vi "Teleop.vi"(10 "Match Info":T1={"Autonomous Elapsed Seconds"=0.0, "TeleOp Elapsed Seconds"=0.0, "Disabled Elapsed Seconds"=0.0, "Visited Autonomous"=FALSE, "Visited TeleOp"=FALSE, "Visited Disabled"=FALSE, "Autonomous Settings"={"Autonomous Style"=enum."Independent", "VI Refnum"=refnum}}, 11 "Call Context":T2) -> ()   [LabVIEW 2015]
doc: "This VI is called for each TeleOp packet received from the DS where the robot is not disabled. It is often used to read from the joysticks and update I/O or to update setpoints for timed control loops. It should complete and return within 20 milliseconds or it may miss DS packets."
uses:
  <vilib>/Rock Robotics/WPI/DriverStation/WPI_DriverStationDerivedRobotMode.ctl
  <vilib>/Rock Robotics/WPI/DriverStation/WPI_DriverStationMatch Info.ctl
  <vilib>/Rock Robotics/WPI/Utilities/WPI_GetSetVariantRefNum.vi
  <vilib>/Rock Robotics/Network Tables/NT Write Boolean Array.vi
  <vilib>/Rock Robotics/Network Tables/NT Write Numeric Array.vi
  <vilib>/Rock Robotics/Network Tables/NT Read Boolean.vi
  <vilib>/Rock Robotics/Network Tables/NT Read Number.vi
panel:
  out "Sample Slider 0":dbl(slide) scale=0.0..5.0
  out "Sample Boolean 1":bool
  out "Sample Boolean 0":bool
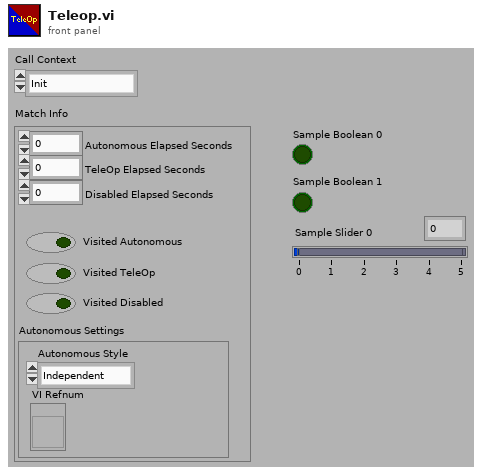
[diagram p1: front panel]
types:
  T1 = typedef "WPI_DriverStationMatch Info.ctl" = cluster{"Autonomous Elapsed Seconds":dbl, "TeleOp Elapsed Seconds":dbl, "Disabled Elapsed Seconds":dbl, "Visited Autonomous":bool, "Visited TeleOp":bool, "Visited Disabled":bool, "Autonomous Settings":cluster{"Autonomous Style":enum16{"Iterative", "Independent"}, "VI Refnum":refnum<vi>}}
  T2 = typedef "WPI_DriverStationDerivedRobotMode.ctl" = enum16{"Init", "Execute", "Stop"}
  T3 = typedef "WPI_JoystickDevRef.ctl" = cluster{"Device":T4}
  T4 = typedef "WPI_JoystickDeviceEnum.ctl" = enum16{"USB 0", "USB 1", "USB 2", "USB 3", "USB 4", "USB 5"}
  T5 = typedef "WPI_RobotDriveDevRef.ctl" = cluster{"DevStatus":errorcluster, "Motors[]":T6[], "Square Inputs":bool, "Max Output":dbl}
  T6 = typedef "WPI_MotorControlDeviceRef.ctl" = cluster{"DeviceStatus":errorcluster, "Type":T7, "PWM":cluster{"PWM Channel":T8, "DeadBand":T9}, "CAN":cluster{"Device Number":u8, "Control Mode":T10, "Semaphore":T11, "Max Vout":dbl, "TalonSRX Control Mode":T12}, "Invert":bool}
  T7 = typedef "WPI_MotorControlType.ctl" = enum16{"PWM", "CAN", "CANTalonSRX"}
  T8 = typedef "FPGA_DIOPWMChannel.ctl" = enum8{"PWM 0", "PWM 1", "PWM 2", "PWM 3", "PWM 4", "PWM 5", "PWM 6", "PWM 7", "PWM 8", "PWM 9", "PWM MXP 0", "PWM MXP 1", "PWM MXP 2", "PWM MXP 3", "PWM MXP 4", "PWM MXP 5", "PWM MXP 6", "PWM MXP 7", "PWM MXP 8", "PWM MXP 9", "Invalid"}
  T9 = typedef "WPI_PWMDeadband.ctl" = cluster{"Name":string, "maxPositivePwm":i32, "minPositivePwm":i32, "centerPwm":i32, "maxNegativePwm":i32, "minNegativePwm":i32, "angularRange":u16}
  T10 = typedef "WPI_CANJaguar_ControlMode.ctl" = enum8{"Percent VBus", "Current", "Speed", "Position", "Voltage"}
  T11 = typedef "Semaphore RefNum" = refnum<k1>
  T12 = typedef "WPI_CANTalonSRX_APIControlMode.ctl" = enum8{"Percent VBus", "Speed", "Position", "Slave", "Unchanged / Invalid", "Voltage Compensation", "Current", "Motion Profile"}
  T13 = typedef "WPI_SwitchDevRef.ctl" = cluster{"DevStatus":errorcluster, "DIO Channel":T14, "CntIndex":T15, "Normally Closed":bool}
  T14 = typedef "FPGA_DIOChannel.ctl" = enum8{"DIO 0", "DIO 1", "DIO 2", "DIO 3", "DIO 4", "DIO 5", "DIO 6", "DIO 7", "DIO 8", "DIO 9", "DIO MXP 0", "DIO MXP 1", "DIO MXP 2", "DIO MXP 3", "DIO MXP 4", "DIO MXP 5", "DIO MXP 6", "DIO MXP 7", "DIO MXP 8", "DIO MXP 9", "DIO MXP 10", "DIO MXP 11", "DIO MXP 12", "DIO MXP 13", "DIO MXP 14", "DIO MXP 15", "Invalid"}
  T15 = typedef "FPGA_CounterCtrSystemIndex.ctl" = enum8{"Ctr 0", "Ctr 1", "Ctr 2", "Ctr 3", "Ctr 4", "Ctr 5", "Ctr 6", "Ctr 7", "Invalid"}
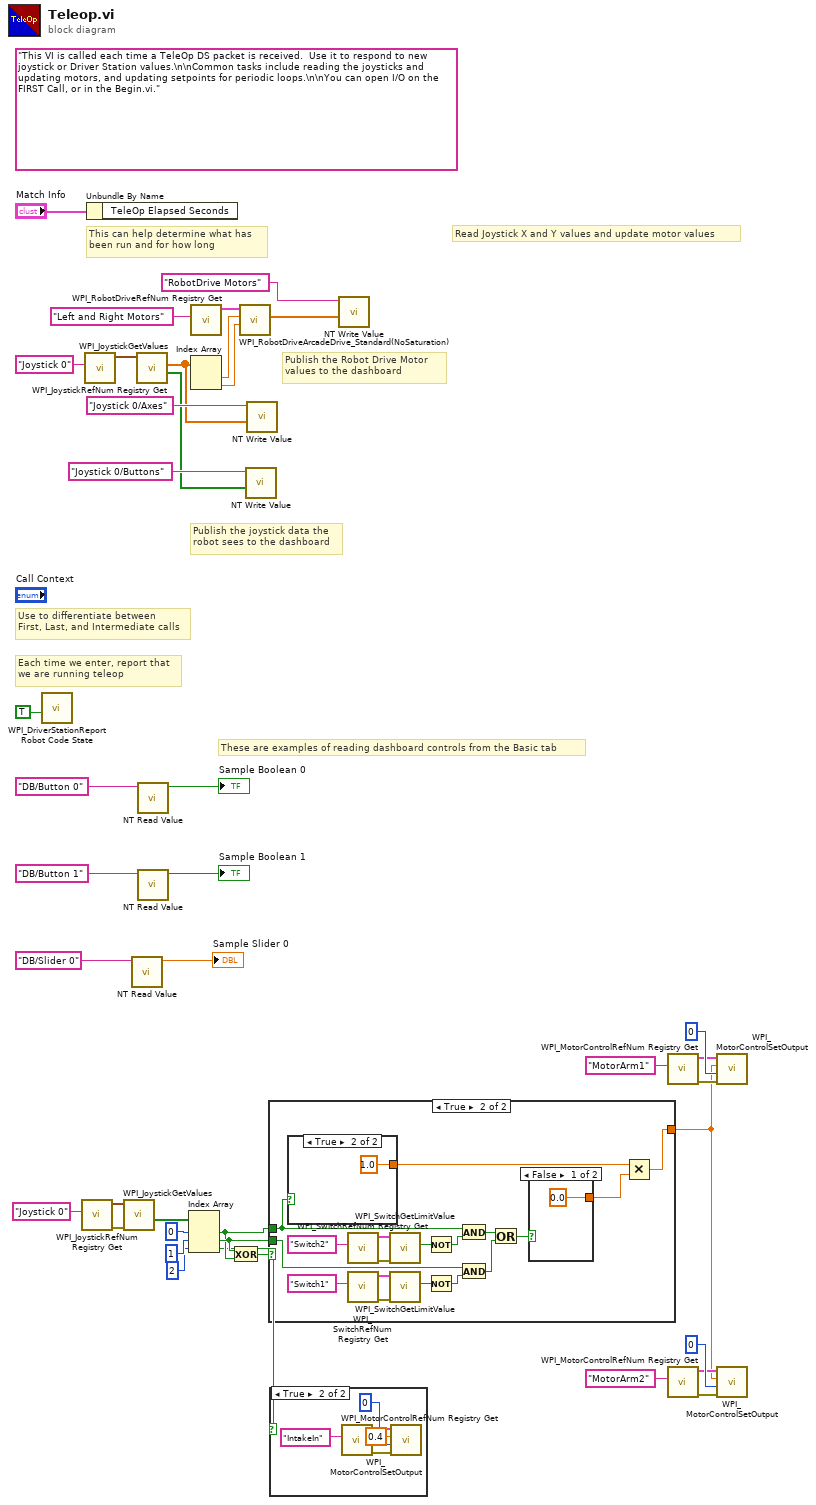
[diagram p0: block diagram]
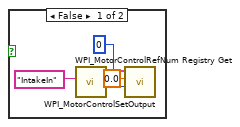
[diagram p2: hidden frame]
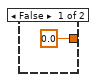
[diagram p3: hidden frame]
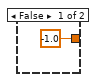
[diagram p4: hidden frame]
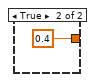
[diagram p5: hidden frame]
diagram:
  (unwired) "This VI is called each time a TeleOp DS packet is received.  Use it to respond to new joystick or Driver Station values.\n\nCommon tasks include reading the joysticks and updating motors, and updating setpoints for periodic loops.\n\nYou can open I/O on the FIRST Call, or in the Begin.vi."
  # "These are examples of reading dashboard controls from the Basic tab"
  # "Publish the Robot Drive Motor\nvalues to the dashboard"
  # "Publish the joystick data the\nrobot sees to the dashboard"
  # "Each time we enter, report that\nwe are running teleop"
  # "Use to differentiate between\nFirst, Last, and Intermediate calls"
  # "This can help determine what has\nbeen run and for how long"
  # "Read Joystick X and Y values and update motor values"
  n1 = call <vilib>:"WPI_DriverStationReport Robot Code State.vi"("TeleOp"=TRUE ("Autonomous")) -> ()  [unwired: 10 in, 1 out]
  n2 = call <vilib>:"WPI_JoystickRefNum Registry Get.vi"("refnum name"="Joystick 0") -> ("error out"=w17:errorcluster, "JoystickDevRef"=w16:T3)  [unwired: 9 in]
  n3 = call <vilib>:"WPI_JoystickRefNum Registry Get.vi"("refnum name"="Joystick 0") -> ("JoystickDevRef"=w35:T3)  [unwired: 1 in, 9 out]
  n4 = Unbundle By Name("Match Info") -> ()  [unwired: 1 out]
  n5 = call <vilib>:"WPI_JoystickGetValues.vi"("error in (no error)"=w17, "JoystickDevRef"=w16) -> ("Buttons"=w15:bool[])  [unwired: 5 in, 4 out]
  n6 = call-poly <vilib>:"NT Read Value.vi"("Name"="DB/Slider 0" ("refnum name")) -> ("Numeric"=→"Sample Slider 0":dbl)  [unwired: 9 in, 1 out]
  n7 = call <vilib>:"WPI_JoystickGetValues.vi"("JoystickDevRef"=w35) -> ("Buttons"=w29:bool[], "Axes"=w30:dbl[])  [unwired: 6 in, 3 out]
  n8 = call-poly <vilib>:"NT Read Value.vi"("Name"="DB/Button 0" ("refnum name")) -> ("Boolean"=→"Sample Boolean 0":bool)  [unwired: 9 in, 1 out]
  n9 = call-poly <vilib>:"NT Read Value.vi"("Name"="DB/Button 1" ("refnum name")) -> ("Boolean"=→"Sample Boolean 1":bool)  [unwired: 9 in, 1 out]
  n10 = Index Array(array=w15, index #1=0 ("index"), index #2=1 ("index"), index #3=2 ("index")) -> (element #1=w10:bool, element #2=w11:bool, element #3=w1:bool)
  n11 = call <vilib>:"WPI_RobotDriveRefNum Registry Get.vi"("refnum name"="Left and Right Motors") -> ("RobotDriveDevRef"=w38:T5)  [unwired: 1 in, 9 out]
  n12 = Index Array(array=w30) -> (element #1=w37:dbl, element #2=w33:dbl)  [unwired: 2 in]
  n13 = Exclusive Or(1:w10, 2:w11) -> (0:w12:bool)
  n14 = call <vilib>:"WPI_RobotDriveArcadeDrive_Standard(NoSaturation).vi"("Y axis value"=w33, "X axis value"=w37, "RobotDriveDevRef"=w38) -> ("Motor Values"=w22:dbl[])  [unwired: 1 in, 7 out]
  n15 = call-poly <vilib>:"NT Write Value.vi"("Boolean Array"=w29, "Name"="Joystick 0/Buttons") -> ()  [unwired: 9 in, 1 out]
  n16 = call-poly <vilib>:"NT Write Value.vi"("Numeric Array"=w30, "Name"="Joystick 0/Axes") -> ()  [unwired: 9 in, 1 out]
  n17 = case shown="True" w12 {
    tunnel: w11 -> [_ w51]
    tunnel: w10 -> [_ w45]
    tunnel: [0.0 w42] -> w4
    frame False {
    }
    frame True {
      n18 = case shown="True" w45 {
        tunnel: [-1.0 1.0] -> w44
        frame False {
        }
        frame True {
        }
      }
      n19 = call <vilib>:"WPI_SwitchRefNum Registry Get.vi"("refnum name"="Switch2") -> ("error out"=w54:errorcluster, "SwitchDevRef"=w55:T13)  [unwired: 9 in]
      n20 = call <vilib>:"WPI_SwitchRefNum Registry Get.vi"("refnum name"="Switch1") -> ("error out"=w56:errorcluster, "SwitchDevRef"=w57:T13)  [unwired: 9 in]
      n21 = call <vilib>:"WPI_SwitchGetLimitValue.vi"("error in (no error)"=w54, "SwitchDevRef"=w55) -> ("Switch Pressed"=w52:bool)  [unwired: 7 in, 2 out]
      n22 = call <vilib>:"WPI_SwitchGetLimitValue.vi"("error in (no error)"=w56, "SwitchDevRef"=w57) -> ("Switch Pressed"=w53:bool)  [unwired: 7 in, 2 out]
      n23 = Not(x=w52) -> (.not. x?=w49:bool)
      n24 = Not(x=w53) -> (.not. x?=w50:bool)
      n25 = And(x=w45, y=w49) -> (x .and. y?=w48:bool)
      n26 = And(x=w51, y=w50) -> (x .and. y?=w47:bool)
      n27 = Or(x=w48, y=w47) -> (x .or. y?=w46:bool)
      n28 = case shown="False" w46 {
        tunnel: [0.0 0.4] -> w43
        frame False {
        }
        frame True {
        }
      }
      n29 = Multiply(x=w44, y=w43) -> (x*y=w42:dbl)
    }
  }
  n30 = case shown="True" w1 {
    frame False {
      n31 = call <vilib>:"WPI_MotorControlRefNum Registry Get.vi"("refnum name"="IntakeIn") -> ("MotorControlDevRef"=w65:T6)  [unwired: 9 in, 1 out]
      n32 = call <vilib>:"WPI_MotorControlSetOutput.vi"("Sync Group / Parameter Slot"=u8 0, "Output"=0.0, "MotorControlDevRef"=w65) -> ()  [unwired: 6 in, 3 out]
    }
    frame True {
      n33 = call <vilib>:"WPI_MotorControlRefNum Registry Get.vi"("refnum name"="IntakeIn") -> ("error out"=w69:errorcluster, "MotorControlDevRef"=w70:T6)  [unwired: 9 in]
      n34 = call <vilib>:"WPI_MotorControlSetOutput.vi"("error in (no error)"=w69, "Sync Group / Parameter Slot"=u8 0, "Output"=0.4, "MotorControlDevRef"=w70) -> ()  [unwired: 5 in, 3 out]
    }
  }
  n35 = call-poly <vilib>:"NT Write Value.vi"("Numeric Array"=w22, "Name"="RobotDrive Motors") -> ()  [unwired: 9 in, 1 out]
  n36 = call <vilib>:"WPI_MotorControlRefNum Registry Get.vi"("refnum name"="MotorArm1") -> ("error out"=w7:errorcluster, "MotorControlDevRef"=w8:T6)  [unwired: 9 in]
  n37 = call <vilib>:"WPI_MotorControlRefNum Registry Get.vi"("refnum name"="MotorArm2") -> ("error out"=w3:errorcluster, "MotorControlDevRef"=w5:T6)  [unwired: 9 in]
  n38 = call <vilib>:"WPI_MotorControlSetOutput.vi"("error in (no error)"=w7, "Sync Group / Parameter Slot"=u8 0, "Output"=w4, "MotorControlDevRef"=w8) -> ()  [unwired: 5 in, 3 out]
  n39 = call <vilib>:"WPI_MotorControlSetOutput.vi"("error in (no error)"=w3, "Sync Group / Parameter Slot"=u8 0, "Output"=w4, "MotorControlDevRef"=w5) -> ()  [unwired: 5 in, 3 out]
